vi "CONSTANT - VI Tester Runner Version.vi"() -> (2 "Version":string="0.1.0")   [LabVIEW 2015, in "G CLI VI Tester.lvlib"]
uses:
  G CLI VI Tester.lvlib
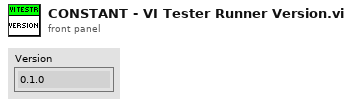
[diagram p1: front panel]
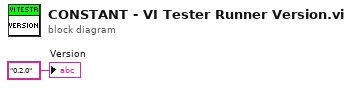
[diagram p0: block diagram]
diagram:
  "Version" <- "0.2.0"
